vi "DecodeInt32.vi"(1 "Data In":u8[](array[numeric])) -> (0 "Data Out":i32[](array[numeric]))   [LabVIEW 2015, in "navX Library v1 (deprecated).lvlib"]
uses:
  navX Library v1 (deprecated).lvlib
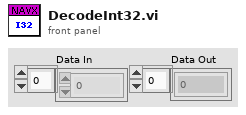
[diagram p1: front panel]
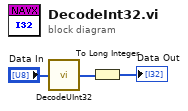
[diagram p0: block diagram]
diagram:
  n1 = call "DecodeUInt32.vi"("Data In"="Data In") -> ("Data Out"=w2:u32[])
  n2 = To Long Integer(number=w2) -> (32bit integer=→"Data Out":i32[])
